vi "get_LBO_set_temp.vi"(8 "error in (no error)":errorcluster, 11 "VISA resource name":refnum<visa-resource-name>) -> (0 "error out":errorcluster, 2 "LBO_set_temp":string, 3 "VISA resource name out":refnum<visa-resource-name>)   [LabVIEW 2013]
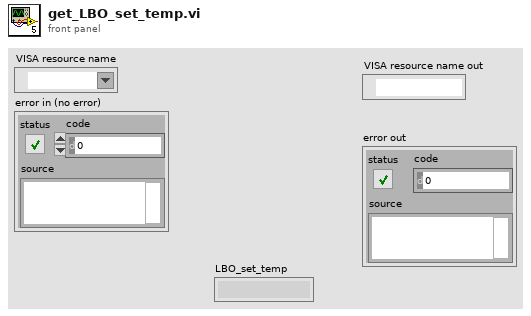
[diagram p1: front panel]
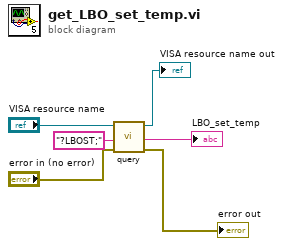
[diagram p0: block diagram]
diagram:
  n1 = call "query.vi"("error in (no error)"="error in (no error)", "write buffer"="?LBOST;", "VISA resource name"="VISA resource name") -> ("error out"=→"error out":errorcluster, "substring"=→"LBO_set_temp":string, "VISA resource name out"=→"VISA resource name out":refnum<visa-resource-name>)  [unwired: 6 in]
